vi "AllAvrStdGraph.vi"() -> ()   [LabVIEW 2023]
panel:
  out "Numeric":dbl
  out "AvrSTDToArr - only six":dbl[](array[numeric])
  in  "const + StdAvr":dbl
  out "Waveform Graph":dbl[][](graph)
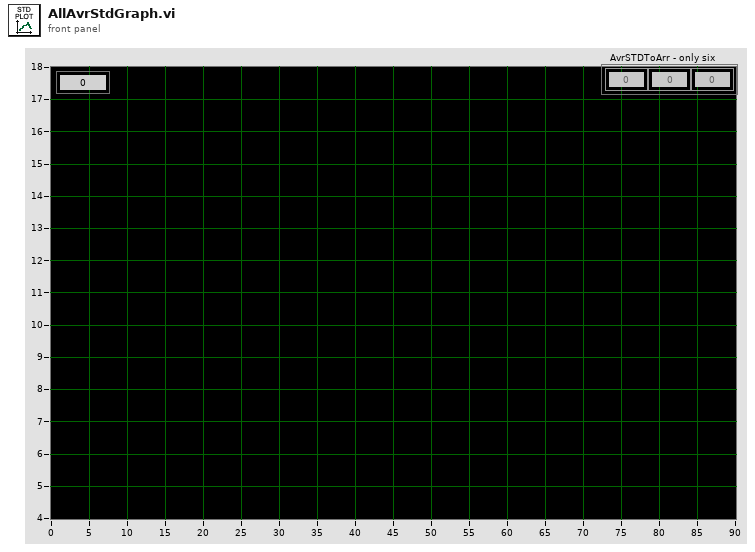
[diagram p1: front panel]
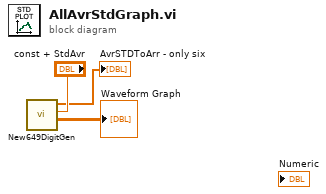
[diagram p0: block diagram]
diagram:
  n1 = call "New649DigitGen.vi"("const + StdAvr"="const + StdAvr") -> ("Waveform Graph"=→"Waveform Graph":dbl[][], "CurrAvrSTDToArr - only six"=→"AvrSTDToArr - only six":dbl[])  [unwired: 8 in, 1 out]
